vi "FIR Windowed Coefficients (obs).vi"(0 "filter type":T2(ring), 1 "high cutoff freq: fh":dbl=0.45 format="%0.2f", 5 "sampling freq: fs":dbl=1.0 format="%0.2f", 7 "taps":i32=25 min=1, 9 "window":T1(ring), 11 "option":enum32{"not scaled", "scaled"}(ring), 12 "low cutoff freq: fl":dbl=0.125 format="%0.2f") -> (4 "FIR Windowed Coefficients":dbl[](array[numeric]), 15 "error":i32)   [LabVIEW 2020, in "NI_AALBase.lvlib"]
doc: "Generates the set of filter coefficients you need to implement a FIR windowed filter."
uses:
  NI_AALBase.lvlib
  AllCosWindow (DBL).vi
  NI_AALPro.lvlib
panel:
  # "This VI is obsolete !!!\nYou should replace this VI in your diagram with the FIR Windowed Coefficients VI.  \n\nNOTE: If you have wired to the window input of this obsolete VI, \n           please be aware that the new FIR Window Coefficients VI has a different\n           window input."
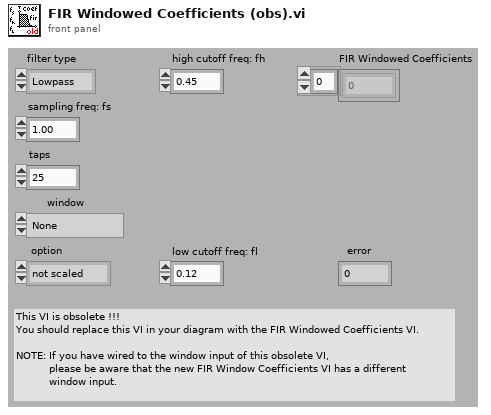
[diagram p1: front panel]
types:
  T1 = enum32{"None", "Hanning", "Hamming", "Triangular", "Blackman", "Exact Blackman", "Blackman-Harris", "Kaiser-Bessel", "Flat Top"}
  T2 = enum32{"Lowpass", "Highpass", "Bandpass", "Bandstop"}
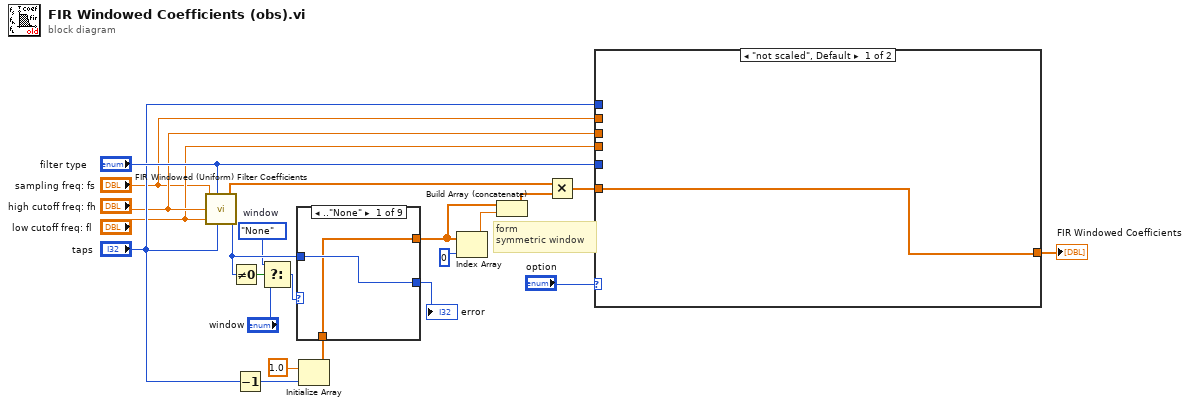
[diagram p0: block diagram]
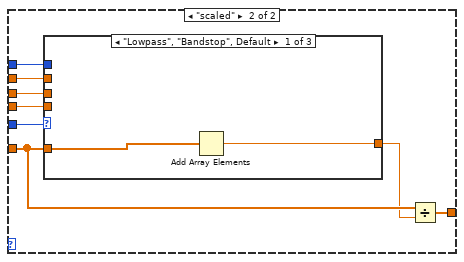
[diagram p2: hidden frame]
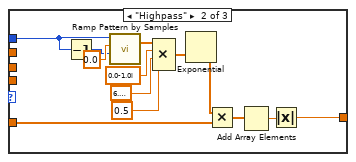
[diagram p3: hidden frame]
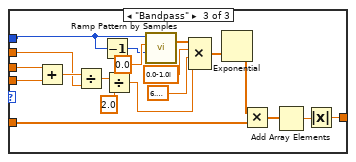
[diagram p4: hidden frame]
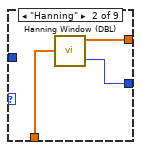
[diagram p5: hidden frame]
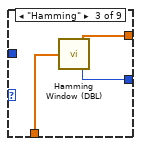
[diagram p6: hidden frame]
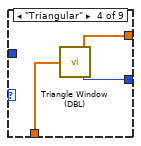
[diagram p7: hidden frame]
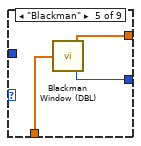
[diagram p8: hidden frame]
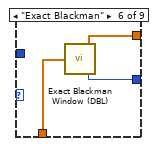
[diagram p9: hidden frame]
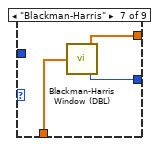
[diagram p10: hidden frame]
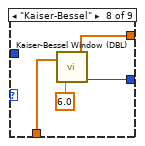
[diagram p11: hidden frame]
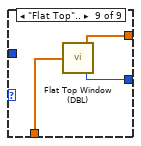
[diagram p12: hidden frame]
diagram:
  w9 = T1."None"  # window
  # "form \nsymmetric window"
  n1 = call "FIR Windowed (Uniform) Filter Coefficients.vi"("sampling freq: fs"="sampling freq: fs", "filter type"="filter type", "high cutoff freq: fh"="high cutoff freq: fh", "low cutoff freq: fl"="low cutoff freq: fl", "taps"="taps") -> ("FIR Coefficients"=w12:dbl[], "error"=w10:i32)
  n2 = Not Equal To 0?(x=w10) -> (x != 0?=w20:bool)
  n3 = Decrement(x="taps") -> (x-1=w17:i32)
  n4 = Select(t=w9, s=w20, f="window") -> (s? t:f=w21:T1)
  n5 = Initialize Array(1.0, w17) -> (w16:dbl[])
  n6 = case shown="..\"None\"" w21 {
    tunnel: [w23 w27 w30 w33 w36 w39 w42 w46 w49] -> w13
    tunnel: [w24 w26 w28 w32 w35 w38 w41 w45 w48] -> w22
    tunnel: w10 -> [w24 _ _ _ _ _ _ _ _]
    tunnel: w16 -> [w23 w25 w29 w31 w34 w37 w40 w44 w47]
    frame .."None" {
    }
    frame "Hanning" {
      n7 = call "Hanning Window (DBL).vi"("X"=w25) -> ("Windowed X"=w27:dbl[], "error"=w26:i32)
    }
    frame "Hamming" {
      n8 = call "Hamming Window (DBL).vi"("X"=w29) -> ("Windowed X"=w30:dbl[], "error"=w28:i32)
    }
    frame "Triangular" {
      n9 = call "Triangle Window (DBL).vi"("X"=w31) -> ("Windowed X"=w33:dbl[], "error"=w32:i32)
    }
    frame "Blackman" {
      n10 = call "Blackman Window (DBL).vi"("X"=w34) -> ("Windowed X"=w36:dbl[], "error"=w35:i32)
    }
    frame "Exact Blackman" {
      n11 = call "Exact Blackman Window (DBL).vi"("X"=w37) -> ("Windowed X"=w39:dbl[], "error"=w38:i32)
    }
    frame "Blackman-Harris" {
      n12 = call "Blackman-Harris Window (DBL).vi"("X"=w40) -> ("Windowed X"=w42:dbl[], "error"=w41:i32)
    }
    frame "Kaiser-Bessel" {
      n13 = call "Kaiser-Bessel Window (DBL).vi"("beta"=6.0, "X"=w44) -> ("error"=w45:i32, "Windowed X"=w46:dbl[])
    }
    frame "Flat Top".. {
      n14 = call "Flat Top Window (DBL).vi"("X"=w47) -> ("Windowed X"=w49:dbl[], "error"=w48:i32)
    }
  }
  "error" <- w22
  n15 = Index Array(array=w13, index=0) -> (element=w14:dbl)
  n16 = Build Array (concatenate)(w13, w14) -> (w11:dbl[])
  n17 = Multiply(x=w12, y=w11) -> (x*y=w3:dbl[])
  n18 = case shown="\"not scaled\", Default" "option" {
    tunnel: "filter type" -> [_ w58]
    tunnel: "taps" -> [_ w57]
    tunnel: "high cutoff freq: fh" -> [_ w56]
    tunnel: "low cutoff freq: fl" -> [_ w55]
    tunnel: "sampling freq: fs" -> [_ w54]
    tunnel: w3 -> [w50 w53]
    tunnel: [w50 w51] -> w2
    frame "not scaled", Default {
    }
    frame "scaled" {
      n19 = case shown="\"Lowpass\", \"Bandstop\", Default" w58 {
        tunnel: w53 -> [w60 w67 w76]
        tunnel: [w59 w64 w74] -> w52
        tunnel: w57 -> [_ w62 w77]
        tunnel: w56 -> [_ _ w92]
        tunnel: w55 -> [_ _ w91]
        tunnel: w54 -> [_ _ w89]
        frame "Lowpass", "Bandstop", Default {
          n20 = Add Array Elements(numeric array=w60) -> (sum=w59:dbl)
        }
        frame "Highpass" {
          n21 = Decrement(x=w62) -> (x-1=w63:i32)
          n22 = call "Ramp Pattern by Samples.vi"("start"=w63, "end"=0.0 ("start"), "samples"=w62) -> ("Ramp Pattern"=w72:dbl[])  [unwired: 7 in, 1 out]
          n23 = Compound Arithmetic op=MULTIPLY(w72, cdb 0.0-1.0i, 6.283185307179586, 0.5 ("start")) -> (w71:cdb[])
          n24 = Exponential(1:w71) -> (0:w68:cdb[])
          n25 = Multiply(x=w68, y=w67) -> (x*y=w66:cdb[])
          n26 = Add Array Elements(numeric array=w66) -> (sum=w65:cdb)
          n27 = Absolute Value(x=w65) -> (abs(x)=w64:dbl)
        }
        frame "Bandpass" {
          n28 = Add(x=w92, y=w91) -> (x+y=w90:dbl)
          n29 = Divide(x=w90, y=w89) -> (x/y=w88:dbl)
          n30 = Decrement(x=w77) -> (x-1=w78:i32)
          n31 = Divide(x=w88, y=2.0) -> (x/y=w75:dbl)
          n32 = call "Ramp Pattern by Samples.vi"("start"=w78, "end"=0.0 ("start"), "samples"=w77) -> ("Ramp Pattern"=w85:dbl[])  [unwired: 7 in, 1 out]
          n33 = Compound Arithmetic op=MULTIPLY(w85, cdb 0.0-1.0i, 6.283185307179586, w75) -> (w84:cdb[])
          n34 = Exponential(1:w84) -> (0:w81:cdb[])
          n35 = Multiply(x=w81, y=w76) -> (x*y=w80:cdb[])
          n36 = Add Array Elements(numeric array=w80) -> (sum=w79:cdb)
          n37 = Absolute Value(x=w79) -> (abs(x)=w74:dbl)
        }
      }
      n38 = Divide(x=w53, y=w52) -> (x/y=w51:dbl[])
    }
  }
  "FIR Windowed Coefficients" <- w2
